vi "Write Vertical Offset.vi"(0 "private data":T1={"GTX2_CHANNEL register map"=refnum, "instruction target"=refnum, "channel measure state"=enum."Uninitialized", "in DFE mode?"=FALSE, "prescale"=0, "rx internal data width"=enum."32 Bit", "active point"={"horizontal offset"=0, "vertical offset"=0}, "ut sign"=enum."Positive", "positive counts"={"sample count"=0, "error count"=0}, "negative counts"={"sample count"=0, "error count"=0}}, 11 "error in":errorcluster) -> (4 "private data out":T1={"GTX2_CHANNEL register map"=refnum, "instruction target"=refnum, "channel measure state"=enum."Uninitialized", "in DFE mode?"=FALSE, "prescale"=0, "rx internal data width"=enum."32 Bit", "active point"={"horizontal offset"=0, "vertical offset"=0}, "ut sign"=enum."Positive", "positive counts"={"sample count"=0, "error count"=0}, "negative counts"={"sample count"=0, "error count"=0}}, 15 "error out":errorcluster)   [LabVIEW 2015, in "niHighSpeedSerial Eye Scan Single Point v1 Host.lvclass"]
doc: "Writes the vertical offset of the point to be measured to the hardware.\n\n<B>Input Parameters</B>\n\n<B>private data</B> is the class private data input into the VI.\n\n<B>private data.GTX2_CHANNEL register map</B> is the GTX2 Channel register map to use.\n\n<B>private data.instruction target</B> is the instruction target to use when communicating with the FPGA.\n\n<B>private data.channel measure state</B> maintains the internal state of the Eye Scan Single Point class.\nenum values: Uninitialized,Initialized,Ready,Request,Wait,Read,Process,Finished\n\n<B>private data.in DFE mode?</B> is true if Eye Scan is configured for DFE Equalization Mode.\n\n<B>private data.prescale</B> controls scaling of the sample count in order to keep the sample count and error count within reasonable precision.\n\n<B>private data.receiver data width</B> is the data width (in bits) of the receiver lane.\nenum values: 16 Bit,20 Bit,32 Bit,40 Bit\n\n<B>private data.active point</B> is the point currently being sampled for errors using Eye Scan.\n\n<B>private data.active point.horizontal offset</B> is the horizontal offset of the active point.\n\n<B>private data.active point.vertical offset</B> is the vertical offset of the active point.\n\n<B>private data.ut sign</B> The untapped threshold sign (positive or negative) currently configured on the point being measured.\nPositive is used when in DFE or LPM Equalization Mode, while Negative is only used in DFE Equalization Mode.\n\n<B>private data.positive counts</B> contains the number of sample and error counts measured using the positive UT Sign.\n\n<B>private data.positive counts.sample count</B> is the positive sample count when using DFE mode, or the entire sample count when using LPM mode.\n\n<B>private data.positive counts.error count</B> is the positive error count when using DFE mode, or the entire error count when using LPM mode.\n\n<B>private data.negative counts</B> contains the number of sample and error counts measured using the negative UT Sign.\n\n<B>private data.negative counts.sample count</B> is the negative sample count when using DFE mode, or unused when using LPM mode.\n\n<B>private data.negative counts.error count</B> is the negative error count when using DFE mode, or unused when using LPM mode.\n\n<B>error in</B> describes error conditions that occur before this node runs. This input provides standard 'error in' functionality.\n\n<B>Output Parameters</B>\n\n<B>private data out</B> is the class private data output from the VI.\n\n<B>private data out.GTX2_CHANNEL register map</B> is the register map to use which represents the GTX2 Channel.\n\n<B>private data out.instruction target</B> is the instruction target to use when communicating with the FPGA.\n\n<B>private data out.channel measure state</B> maintains the internal state of the Eye Scan Single Point class.\nenum values: Uninitialized,Initialized,Ready,Request,Wait,Read,Process,Finished\n\n<B>private data out.in DFE mode?</B> is true if Eye Scan is configured for DFE Equalization Mode.\n\n<B>private data out.prescale</B> controls scaling of the sample count in order to keep the sample count and error count within reasonable precision.\n\n<B>private data out.receiver data width</B> is the data width (in bits) of the receiver lane.\nenum values: 16 Bit,20 Bit,32 Bit,40 Bit\n\n<B>private data out.active point</B> is the point currently being sampled for errors using Eye Scan.\n\n<B>private data out.active point.horizontal offset</B> is the horizontal offset of the active point.\n\n<B>private data out.active point.vertical offset</B> is the vertical offset of the active point.\n\n<B>private data out.ut sign</B> contains the number of sample and error counts measured using the positive UT Sign.\nenum values: Positive,Negative\n\n<B>private data out.positive counts</B> contains the number of sample and error counts measured using the positive UT Sign.\n\n<B>private data out.positive counts.sample count</B> is the positive sample count when using DFE mode, or the entire sample count when using LPM mode.\n\n<B>private data out.positive counts.error count</B> is the positive error count when using DFE mode, or the entire error count when using LPM mode.\n\n<B>private data out.negative counts</B> contains the number of sample and error counts measured using the negative UT Sign.\n\n<B>private data out.negative counts.sample count</B> is the negative sample count when using DFE mode, or the entire sample count when using LPM mode.\n\n<B>private data out.negative counts.error count</B> is the negative error count when using DFE mode, or the entire error count when using LPM mode.\n\n<B>error out</B> contains error information. This output provides standard 'error out' functionality."
uses:
  <instrlib>/niHighSpeedSerial/Eye Scan/v1/Host/Impl/Single Point/niHighSpeedSerial Eye Scan Single Point v1 Host.lvclass
  <instrlib>/niHighSpeedSerial/Eye Scan/v1/Host/Impl/Single Point/Private/Private Data.ctl
  <instrlib>/niHighSpeedSerial/Register Maps/Xilinx/v1/Host/GTX2_CHANNEL v1 Host.llb/GTX2_CHANNEL Register Map.lvclass
  <instrlib>/_niInstr/Instruction Framework/v1/Host/Instruction Target/niInstr Instruction Target v1 Host.lvclass
  <instrlib>/niHighSpeedSerial/Eye Scan/v1/Host/Impl/Single Point/Private/Channel Measure State.ctl
  <instrlib>/niHighSpeedSerial/Eye Scan/v1/Host/Common/Public/Data Width.ctl
  <instrlib>/niHighSpeedSerial/Eye Scan/v1/Host/Common/Public/Point Offsets.ctl
  <instrlib>/niHighSpeedSerial/Register Maps/Xilinx/v1/Host/GTX2_CHANNEL v1 Host.llb/ESVertOffsetSign.ctl
  <instrlib>/niHighSpeedSerial/Eye Scan/v1/Host/Impl/Single Point/Private/Counts.ctl
  <instrlib>/niHighSpeedSerial/Register Maps/Xilinx/v1/Host/GTX2_CHANNEL v1 Host.llb/GTX2_CHANNEL Register Map.lvclass/GTX2_CHANNEL Register Map.ctl
  <instrlib>/niHighSpeedSerial/Register Maps/Xilinx/v1/Host/GTX2_CHANNEL v1 Host.llb/Read ES_VERT_OFFSET.vi
  <instrlib>/niHighSpeedSerial/Register Maps/Xilinx/v1/Host/GTX2_CHANNEL v1 Host.llb/Write ES_VERT_OFFSET.vi
  <instrlib>/niHighSpeedSerial/Register Maps/Xilinx/v1/Host/GTX2_CHANNEL v1 Host.llb/Decode Register to Address.vi
  <instrlib>/_niInstr/Instruction Framework/v1/Host/Instruction Target/Public/Context Read.vi
  <instrlib>/_niInstr/Instruction Framework/v1/Host/Instruction Target/Public/Context Write.vi
  <instrlib>/niHighSpeedSerial/Register Maps/Xilinx/v1/Host/GTX2_CHANNEL v1 Host.llb/GTX2_CHANNEL v1 Host.lvlib
  <instrlib>/niHighSpeedSerial/Eye Scan/v1/Host/Common/niHighSpeedSerial Eye Scan Common v1 Host.lvlib
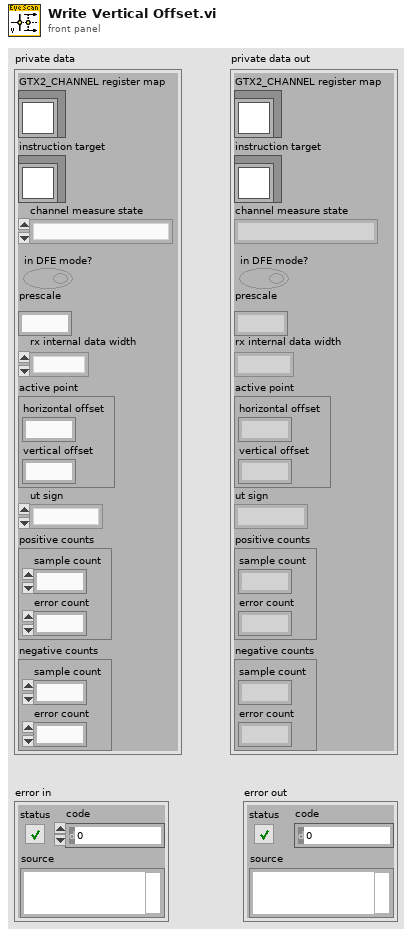
[diagram p1: front panel]
types:
  T1 = typedef "niHighSpeedSerial Eye Scan Single Point v1 Host.lvclass/Private Data.ctl" = cluster{"GTX2_CHANNEL register map":refnum<class "GTX2_CHANNEL Register Map.lvclass">, "instruction target":refnum<class "niInstr Instruction Target v1 Host.lvclass">, "channel measure state":T2, "in DFE mode?":bool, "prescale":u8, "rx internal data width":T3, "active point":T4, "ut sign":T5, "positive counts":T6, "negative counts":T6}
  T2 = typedef "niHighSpeedSerial Eye Scan Single Point v1 Host.lvclass/Channel Measure State.ctl" = enum16{"Uninitialized", "Initialized", "Ready", "Request", "Wait", "Read", "Process", "Finished"}
  T3 = typedef "niHighSpeedSerial Eye Scan Common v1 Host.lvlib/Data Width.ctl" = enum16{"16 Bit", "20 Bit", "32 Bit", "40 Bit"}
  T4 = typedef "niHighSpeedSerial Eye Scan Common v1 Host.lvlib/Point Offsets.ctl" = cluster{"horizontal offset":i16, "vertical offset":i8}
  T5 = typedef "GTX2_CHANNEL v1 Host.lvlib/ESVertOffsetSign.ctl" = enum8{"Positive", "Negative"}
  T6 = typedef "niHighSpeedSerial Eye Scan Single Point v1 Host.lvclass/Counts.ctl" = cluster{"sample count":u64, "error count":u16}
  T7 = typedef "GTX2_CHANNEL v1 Host.lvlib/ES_VERT_OFFSET.ctl" = cluster{"ES_VERT_OFFSET_MAGNITUDE":u8, "ES_VERT_OFFSET_SIGN":T5, "ES_VERT_OFFSET_UT_SIGN":T5, "RESERVED":u8, "ES_PRESCALE":u8}
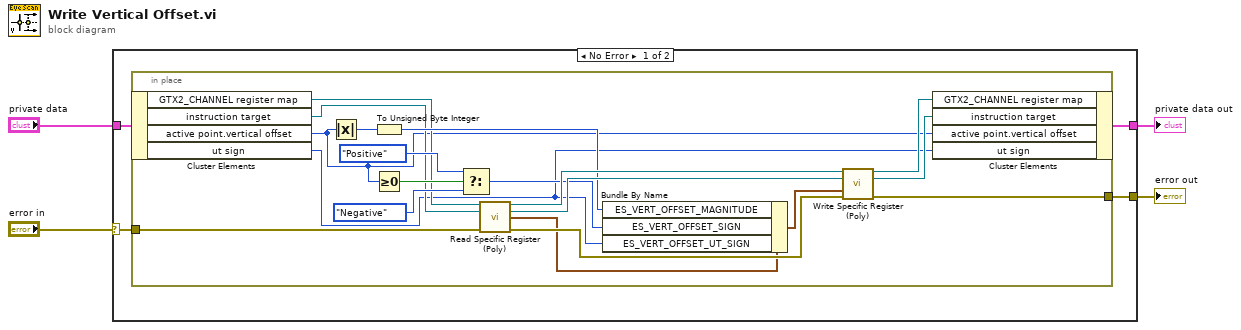
[diagram p0: block diagram]
diagram:
  n1 = case shown="No Error" "error in" {
    selector: "error in" -> [w8 w29]
    tunnel: [w5 w29] -> w4
    tunnel: "private data" -> [w7 w28]
    tunnel: [w6 w28] -> w1
    frame No Error {
      n2 = in-place {
        in-place-border: w8 -> [w27]
        in-place-border: [w26] -> w5
        n3 = in-place-cluster #1(w7) -> ("GTX2_CHANNEL register map"=w14:refnum<class "GTX2_CHANNEL Register Map.lvclass">, "instruction target"=w13:refnum<class "niInstr Instruction Target v1 Host.lvclass">, "active point.vertical offset"=w10:i8, "ut sign"=w9:T5)
        n4 = Absolute Value(x=w10) -> (abs(x)=w20:i8)
        n5 = To Unsigned Byte Integer(number=w20) -> (unsigned 8bit integer=w19:u8)
        n6 = Greater Or Equal To 0?(x=w10) -> (x >= 0?=w18:bool)
        n7 = Select(t=ESVertOffsetSign."Positive" ("ES_VERT_OFFSET_SIGN"), s=w18, f=ESVertOffsetSign."Negative") -> (s? t:f=w16:T5)
        n8 = call-poly <instrlib>:"Read Specific Register (Poly).vi"("gtx2_channel register map object in"=w14, "instruction target in"=w13, "error in"=w27) -> ("gtx2_channel register map object out"=w24:refnum<class "GTX2_CHANNEL Register Map.lvclass">, "instruction target out"=w25:refnum<class "niInstr Instruction Target v1 Host.lvclass">, "ES_VERT_OFFSET"=w22:T7, "error out"=w23:errorcluster)  [unwired: 9 in]
        n9 = Bundle By Name(cluster=w22, "ES_VERT_OFFSET_MAGNITUDE"=w19, "ES_VERT_OFFSET_SIGN"=w16, "ES_VERT_OFFSET_UT_SIGN"=w9) -> (w21:T7)
        n10 = call-poly <instrlib>:"Write Specific Register (Poly).vi"("gtx2_channel register map object in"=w24, "instruction target in"=w25, "ES_VERT_OFFSET"=w21, "error in"=w23) -> ("gtx2_channel register map object out"=w12:refnum<class "GTX2_CHANNEL Register Map.lvclass">, "instruction target out"=w11:refnum<class "niInstr Instruction Target v1 Host.lvclass">, "error out"=w26:errorcluster)  [unwired: 9 in]
        n11 = in-place-cluster #1("GTX2_CHANNEL register map"=w12, "instruction target"=w11, "active point.vertical offset"=w10, "ut sign"=w9) -> (w6:T1)
      }
    }
    frame Error {
    }
  }
  "error out" <- w4
  "private data out" <- w1
